vi "Switch_heater_wait.vi"(1 "T-Start":timestamp, 2 "Switch waiting time":dbl format="%#_13g") -> ()   [LabVIEW 2016]
uses:
  Global/Global Variables/Data_Display_global.vi
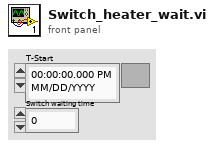
[diagram p1: front panel]
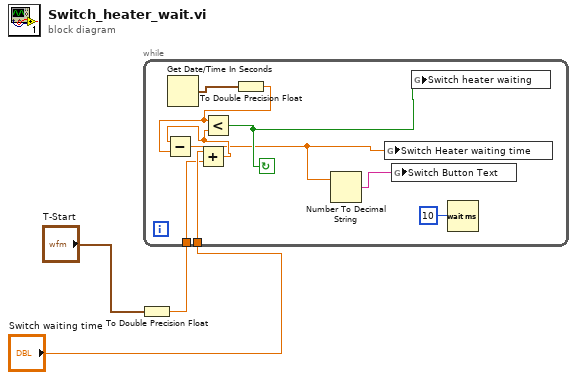
[diagram p0: block diagram]
diagram:
  n1 = To Double Precision Float(number="T-Start") -> (double precision float=w3:dbl)
  n2 = while {
    tunnel: "Switch waiting time" -> [w12]
    tunnel: w3 -> [w11]
    stop <- w9 continue-if-true
    n3 = Get Date/Time In Seconds() -> (seconds since 1Jan1904=w8:timestamp)
    n4 = Add(x=w12, y=w11) -> (x+y=w10:dbl)
    n5 = To Double Precision Float(number=w8) -> (double precision float=w7:dbl)
    n6 = Subtract(x=w10, y=w7) -> (x-y=w5:dbl)
    n7 = Less?(x=w7, y=w10) -> (x < y?=w9:bool)
    n8 = Number To Decimal String(number=w5) -> (decimal integer string=w4:string)  [unwired: 1 in]
    n9 = global write "Data_Display_global.vi" "Switch Heater waiting time"(w5) -> ()
    n10 = global write "Data_Display_global.vi" "Switch Button Text"(w4) -> ()
    n11 = global write "Data_Display_global.vi" "Switch heater waiting"(w9) -> ()
    n12 = Wait (ms)(milliseconds to wait=10) -> ()  [unwired: 1 out]
  }
